vi "Enable Output.vi"(8 "error in (no error)":errorcluster, 10 "Enable Output (F: False)":bool, 11 "VISA resource name":refnum<visa-resource-name>) -> (0 "error out":errorcluster, 3 "VISA resource name out":refnum<visa-resource-name>)   [LabVIEW 2015, in "BK Precision 983X Series.lvlib"]
doc: "Enables or Disables the output."
uses:
  <instrlib>/BK Precision 983X Series/BK Precision 983X Series.lvlib
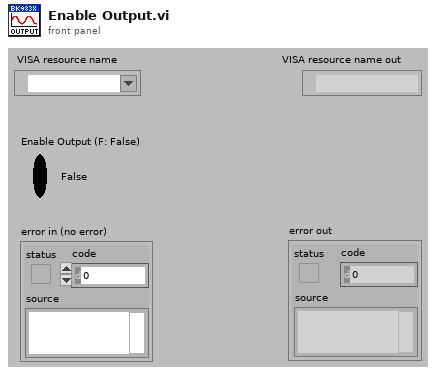
[diagram p1: front panel]
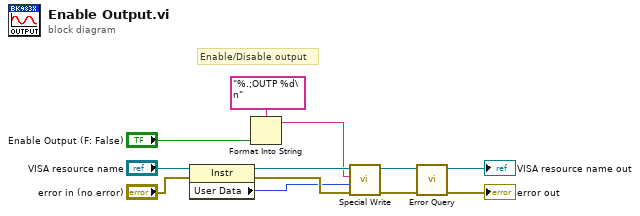
[diagram p0: block diagram]
diagram:
  # "Enable/Disable output"
  n1 = property class="Instr"(reference="VISA resource name", error in="error in (no error)") -> (reference out=w6:refnum<visa-resource-name>, error out=w5:errorcluster, "User Data"=w4:u32)
  n2 = Format Into String(format string="%.;OUTP %d\n", "Enable Output (F: False)") -> (resulting string=w3:string)  [unwired: 2 in, 1 out]
  n3 = call <instrlib>:"Special Write.vi"("error in (no error)"=w5, "Delay (0 ms)"=w4, "Input String"=w3, "VISA resource name"=w6) -> ("error out"=w1:errorcluster, "VISA resource name out"=w2:refnum<visa-resource-name>)  [unwired: 6 in]
  n4 = call <instrlib>:"Error Query.vi"("error in (no error)"=w1, "VISA resource name"=w2) -> ("error out"=→"error out":errorcluster, "VISA resource name out"=→"VISA resource name out":refnum<visa-resource-name>)  [unwired: 6 in, 2 out]
